vi "Reference_Action_SLM.vi"(0 "VI Ref IN":refnum<vi>, 2 "Action":u16(ring) items=["Read", "Initialize"], 9 "Control Name":string) -> (4 "VI Reference":refnum<vi>, 8 "Ref OUT":refnum<vi>, 13 "Array":string[](array[string]))   [LabVIEW 2014]
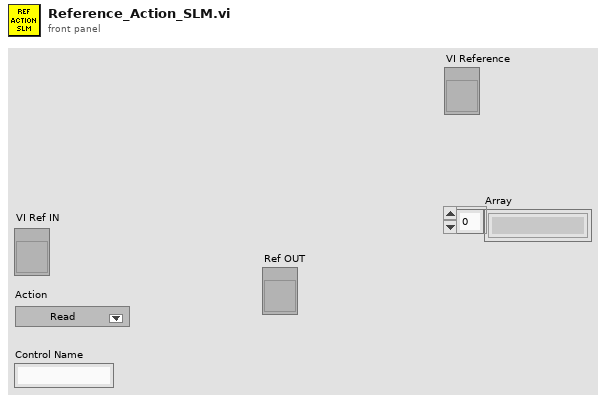
[diagram p1: front panel]
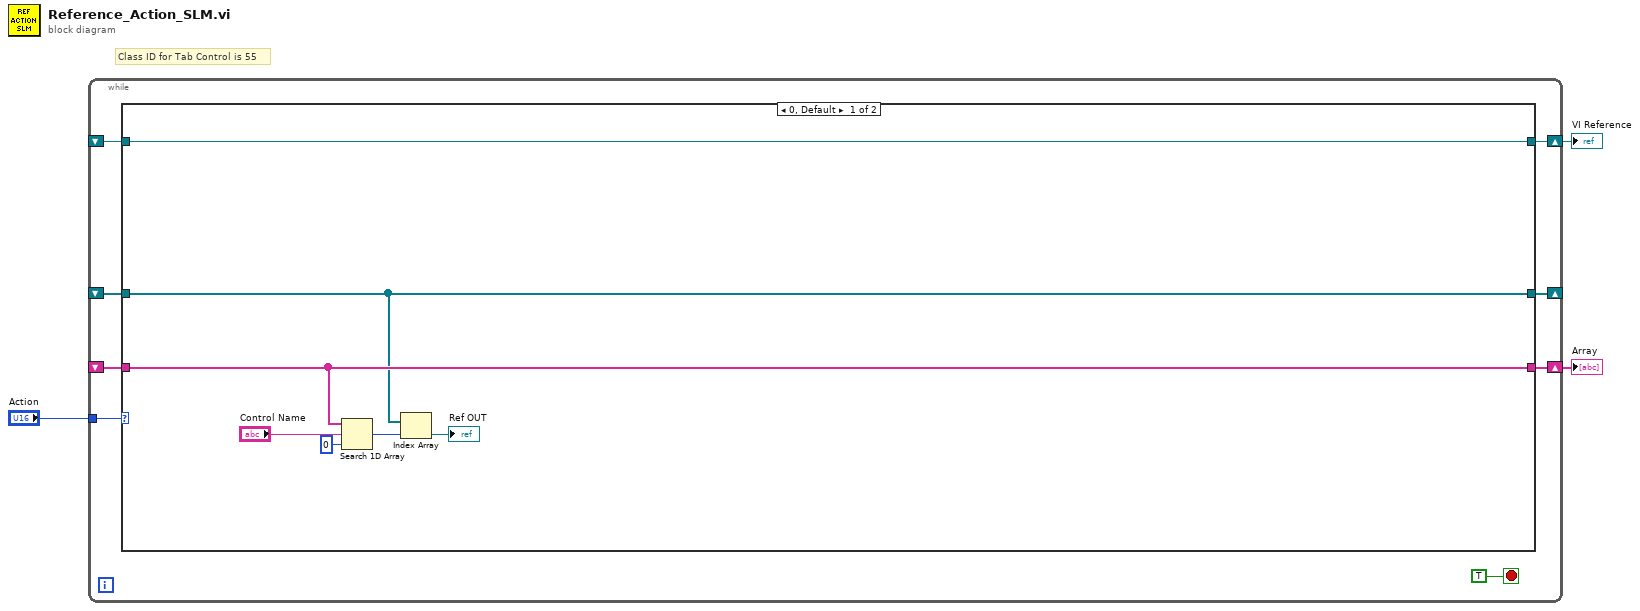
[diagram p0: block diagram]
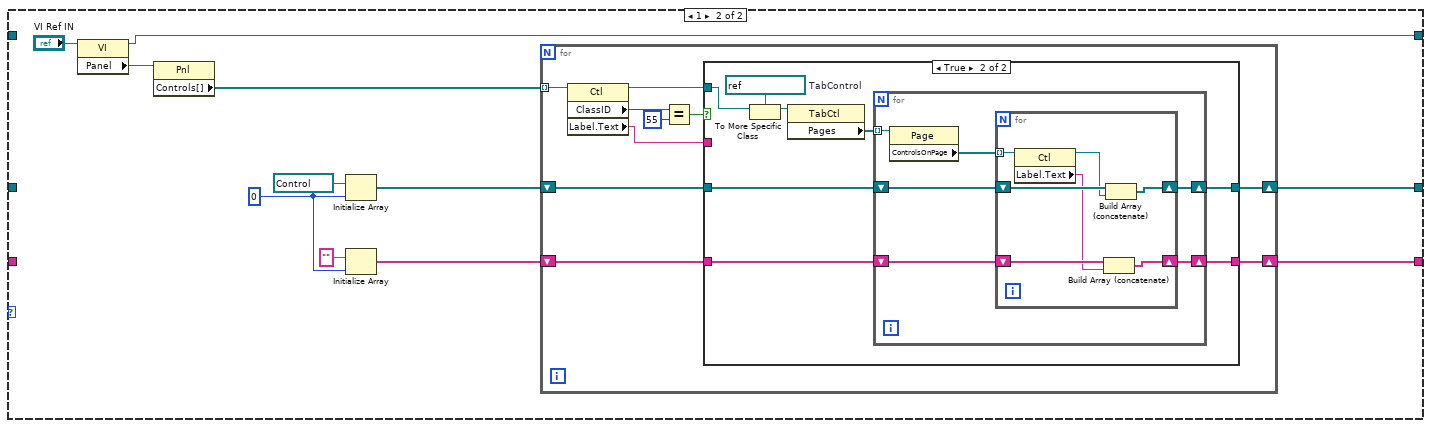
[diagram p2: hidden frame]
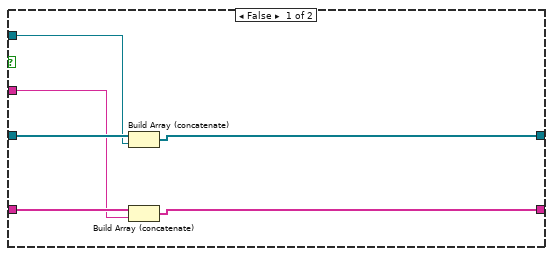
[diagram p3: hidden frame]
diagram:
  # "Class ID for Tab Control is 55"
  n1 = while {
    shift-right: [w10] -> _
    shift-left: _ -> [w7]
    shift-right: [w9] -> w1
    shift-left: _ -> [w6]
    tunnel: "Action" -> [w8]
    shift-right: [w5] -> w2
    shift-left: _ -> [w4]
    stop <- TRUE stop-if-true
    n2 = case shown="0, Default" w8 {
      tunnel: [w14 w21] -> w10
      tunnel: [w18 w27] -> w9
      tunnel: w7 -> [w14 _]
      tunnel: w6 -> [w18 _]
      tunnel: [w12 w20] -> w5
      tunnel: w4 -> [w12 _]
      frame 0, Default {
        n3 = Search 1D Array(1D array=w18, element="Control Name", start index (0)=0) -> (index of element=w15:i32)
        n4 = Index Array(array=w14, index=w15) -> (element=→"Ref OUT":refnum<vi>)
      }
      frame 1 {
        w24 = 0 ("dimension size")
        n5 = property class="VI"(reference="VI Ref IN") -> (reference out=w20:refnum<vi>, "Panel"=w29:refnum<vi>)  [unwired: 1 in, 1 out]
        n6 = property class="Pnl"(reference=w29) -> ("Controls[]"=w28:refnum<vi>[])  [unwired: 1 in, 2 out]
        n7 = Initialize Array(refnum<vi> refnum ("reference out"), w24) -> (w23:refnum<vi>[])
        n8 = Initialize Array("", w24) -> (w22:string[])
        n9 = for {
          shift-right: [w31] -> w21
          shift-left: w23 -> [w33]
          shift-right: [w30] -> w27
          shift-left: w22 -> [w32]
          tunnel: w28 -> [w39] mode=indexing
          n10 = property class="Ctl"(reference=w39) -> (reference out=w35:refnum<vi>, "ClassID"=w38:u32, "Label.Text"=w34:string)  [unwired: 1 in, 1 out]
          n11 = Equal?(x=w38, y=u32 55) -> (x = y?=w36:bool)
          n12 = case shown="True" w36 {
            tunnel: w35 -> [w43 w51]
            tunnel: w34 -> [w42 _]
            tunnel: w33 -> [w45 w49]
            tunnel: w32 -> [w44 w48]
            tunnel: [w41 w47] -> w31
            tunnel: [w40 w46] -> w30
            frame False {
              n13 = Build Array (concatenate)(w45, w43) -> (w41:refnum<vi>[])
              n14 = Build Array (concatenate)(w44, w42) -> (w40:string[])
            }
            frame True {
              w53 = refnum<vi> refnum  # TabControl
              n15 = To More Specific Class(target class=w53, reference=w51) -> (specific class reference=w52:refnum<vi>)  [unwired: 1 in, 1 out]
              n16 = property class="TabCtl"(reference=w52) -> ("Pages"=w50:refnum<vi>[])  [unwired: 1 in, 2 out]
              n17 = for {
                tunnel: w50 -> [w59] mode=indexing
                shift-right: [w55] -> w47
                shift-left: w49 -> [w57]
                shift-right: [w54] -> w46
                shift-left: w48 -> [w56]
                n18 = property class="Page"(reference=w59) -> ("ControlsOnPage"=w58:refnum<vi>[])  [unwired: 1 in, 2 out]
                n19 = for {
                  tunnel: w58 -> [w66] mode=indexing
                  shift-right: [w61] -> w55
                  shift-left: w57 -> [w64]
                  shift-right: [w60] -> w54
                  shift-left: w56 -> [w65]
                  n20 = property class="Ctl"(reference=w66) -> (reference out=w63:refnum<vi>, "Label.Text"=w62:string)  [unwired: 1 in, 1 out]
                  n21 = Build Array (concatenate)(w65, w62) -> (w60:string[])
                  n22 = Build Array (concatenate)(w64, w63) -> (w61:refnum<vi>[])
                }
              }
            }
          }
        }
      }
    }
  }
  "VI Reference" <- w2
  "Array" <- w1
